vi "De Interleave FPGA Data.vi"(10 "Number of Interleaved Channels":u32=3, 11 "Interleaved Data":dbl[](array[numeric])=[1.0, 2.0, 3.0, 4.0, 5.0, 6.0, 7.0, 8.0, 9.0, 10.0]) -> (3 "De-Interleaved Channel Data":dbl[][](array[numeric])=[[2.0, 5.0, 8.0], [3.0, 6.0, 9.0], [1.0, 4.0, 7.0]])   [LabVIEW 2018]
doc: "This VI demonstrates how to de-interleave a 1D array that contains data of multiple channels. The output will be a 2D array where each row contains values of one channel. If the quotient of Interleaved Data values and Number of Channels is not an integer, remaining values are ignored."
panel:
  out "subarray":dbl[](array[numeric])
  # "Overview: This VI demonstrates how to de-interleave a 1D array that contains data of multiple channels.\n                    The output will be a 2D array where each row contains values of one channel.\n                    If the quotient of Interleaved Data values and Number of Channels is not an integer, remaining values are ignored.\nRequirements: LabVIEW Base Development System 2012 (or compatible)\n\nInstructions: \n1. Use default values for \"Number of Interleaved Channels\" and \"Interleaved Data\" or enter your own values.\n2. Run VI"
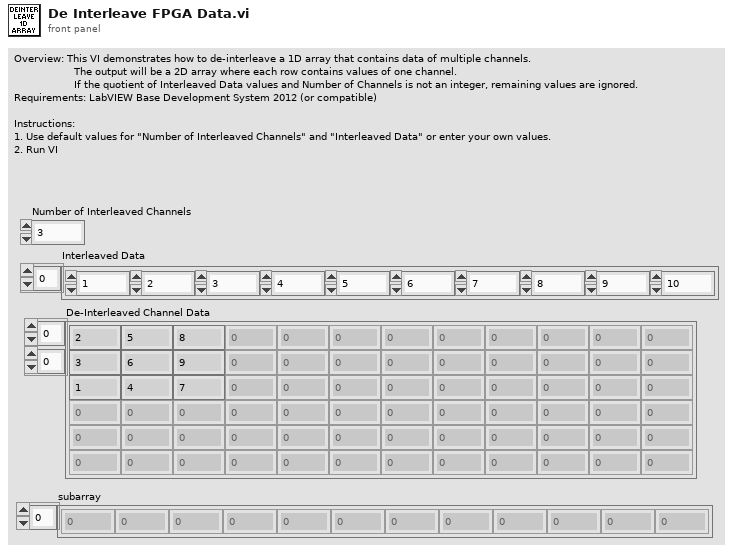
[diagram p1: front panel]
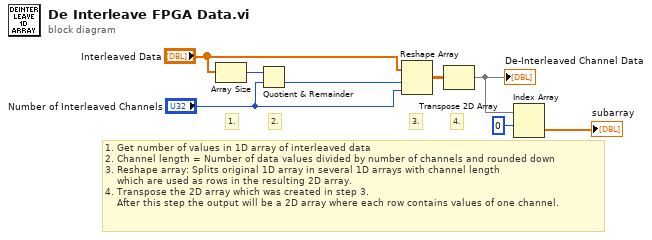
[diagram p0: block diagram]
diagram:
  # "1. Get number of values in 1D array of interleaved data\n2. Channel length = Number of data values divided by number of channels and rounded down\n3. Reshape array: Splits original 1D array in several 1D arrays with channel length\n    which are used as rows in the resulting 2D array.\n4. Transpose the 2D array which was created in step 3. \n    After this step the output will be a 2D array where each row contains values of one channel."
  # "4."
  # "3."
  # "2."
  # "1."
  n1 = Array Size(array="Interleaved Data") -> (size(s)=w8:i32)
  n2 = Quotient & Remainder(x=w8, y="Number of Interleaved Channels") -> (floor(x/y)=w7:u32)  [unwired: 1 out]
  n3 = Reshape Array("Interleaved Data", w7, "Number of Interleaved Channels") -> (w5:dbl[][])
  n4 = Transpose 2D Array(2D array=w5) -> (transposed array=w3:dbl[][])
  "De-Interleaved Channel Data" <- w3
  n5 = Index Array(array=w3, index (row)=0) -> (element=→"subarray":dbl[])  [unwired: 1 in]
